vi "Data Source RW.vi"(6 "section":string="info", 7 "Operate":enum16{"Read", "Write"}(ring), 8 "Error In":errorcluster, 10 "Source Path":path caption="配置文件的路径", 11 "Data Type In":T1) -> (0 "Error Out":errorcluster, 1 "Data":string[](array[string]), 2 "Name":string[](array[string]), 3 "Data Type Out":T1)   [LabVIEW 2020]
uses:
  0007 Controls/005 Data Source Type.ctl
  c7fef91f-c7a3-4238-a59e-1a6f217abd33.vi
  <vilib>/Utility/config.llb/Open Config Data.vi
  <vilib>/Utility/config.llb/Read Key.vi
  <vilib>/Utility/config.llb/Read Key (String).vi
  <vilib>/Utility/config.llb/Write Key.vi
  <vilib>/Utility/config.llb/Write Key (String).vi
  <vilib>/Utility/config.llb/Close Config Data.vi
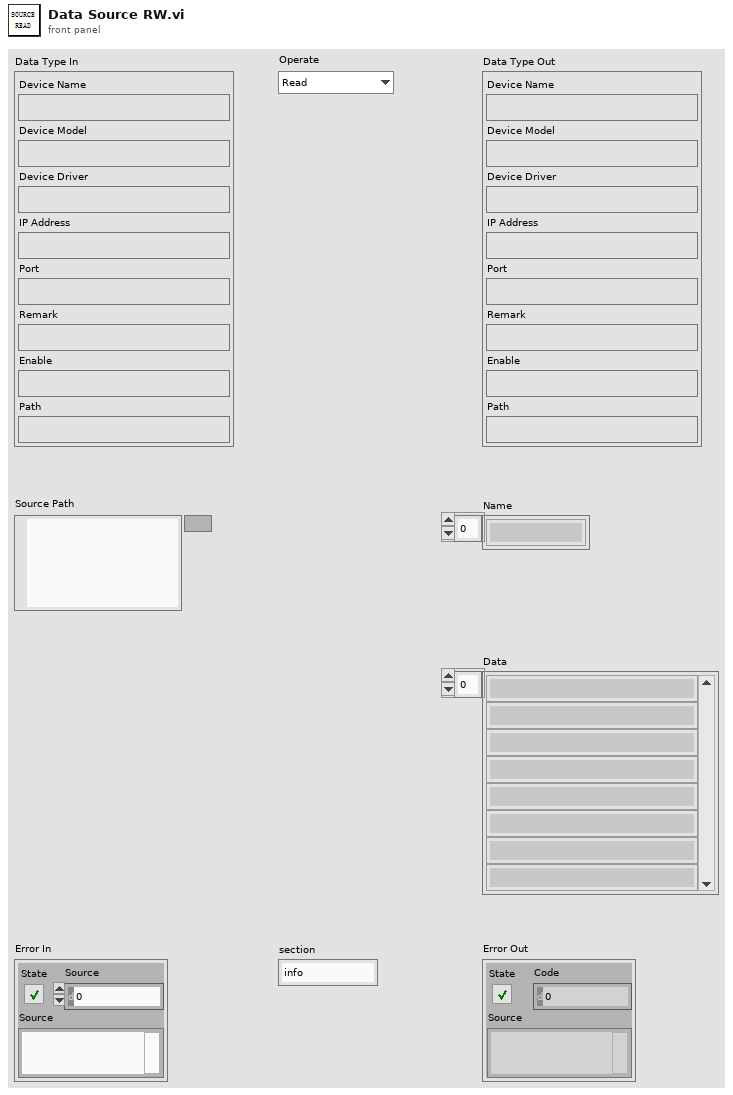
[diagram p1: front panel]
types:
  T1 = typedef "005 Data Source Type.ctl" = cluster{"Device Name":string, "Device Model":string, "Device Driver":string, "IP Address":string, "Port":string, "Remark":string, "Enable":string, "Path":string}
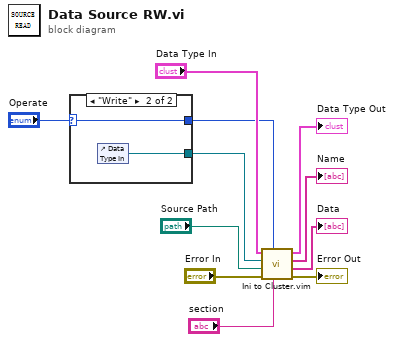
[diagram p0: block diagram]
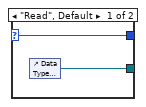
[diagram p2: hidden frame]
diagram:
  n1 = case shown="\"Write\"" "Operate" {
    selector: "Operate" -> [w13 w15]
    tunnel: [w12 w14] -> w3
    tunnel: [w13 w15] -> w2
    frame "Read", Default {
      n2 = control-ref of="Data Type Out"() -> (w12:refnum<vi>)
    }
    frame "Write" {
      n3 = control-ref of="Data Type In"() -> (w14:refnum<vi>)
    }
  }
  n4 = call "Ini to Cluster.vim"("section"="section", "Operate"=w2, "Error In"="Error In", "Source Path"="Source Path", "Cluster Ref In"=w3, "Cluster Type In"="Data Type In") -> ("Error Out"=→"Error Out":errorcluster, "Data"=→"Data":string[], "Name"=→"Name":string[], "Cluster Out"=→"Data Type Out":T1)  [unwired: 2 in]
